vi "OdomLaserSubscriber.vi"() -> (0 "Odom Error Out":errorcluster)   [LabVIEW 2014]
doc: "Reads in the odometry from the Turtlebot"
uses:
  <vilib>/Tufts CEEO ROS for LabVIEW Software/ROS/Code/Console/Servers/ServerSubs/TopicDef.ctl
  <vilib>/Tufts CEEO ROS for LabVIEW Software/ROS/Code/SubVIs/_ROSDirection.ctl
panel:
  out "Scan Details":T1
  in  "?":bool
  in  "Update Time (ms)":u32
  out "Laser Scan Plot (in Husky Frame)":cluster{dbl[], dbl[]}(graph)
  out "Scan Error Out":errorcluster
  out "2D Pose":cluster{"x":dbl, "y":dbl}
  out "Husky Pose Plot":cluster{"X":dbl, "Y":dbl}[](graph)
  out "Husky EKF Odometry":T2
  in  "Stop Subscribing":bool
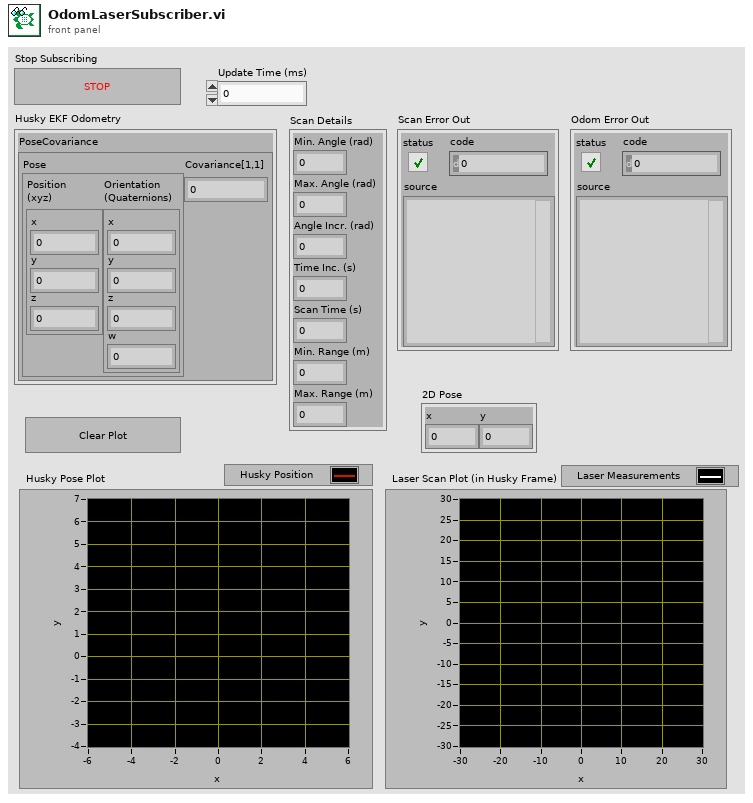
[diagram p1: front panel]
types:
  T1 = cluster{"Min. Angle (rad)":dbl, "Max. Angle (rad)":dbl, "Angle Incr. (rad)":dbl, "Time Inc. (s)":dbl, "Scan Time (s)":dbl, "Min. Range (m)":dbl, "Max. Range (m)":dbl}
  T2 = cluster{"PoseCovariance":cluster{"Pose":cluster{"Position\n(xyz)":cluster{"x":dbl, "y":dbl, "z":dbl}, "Orientation\n(Quaternions)":cluster{"x":dbl, "y":dbl, "z":dbl, "w":dbl}}, "Covariance[1,1]":dbl}}
  T3 = typedef "TopicDef.ctl" = cluster{"Topic":string, "Type":string, "Action":T4, "Update (ms)":u16, "queue size":u16}
  T4 = typedef "_ROSDirection.ctl" = enum16{"Node", "Publisher", "Subscriber", "ServiceClient", "ServiceProvider"}
  T5 = typedef "_ROSControl.ctl" = cluster{"topic port":u16, "Node":string, "topic":string, "type":string, "node port":u16, "error ":errorcluster, "Direction":T4, "Update (ms)":u16, "FIFO size":u16}
  T6 = cluster{"PoseCovariance":cluster{"Pose":cluster{"Point":cluster{"x":dbl, "y":dbl, "z":dbl}, "Quaternion":cluster{"x":dbl, "y":dbl, "z":dbl, "w":dbl}}, "Covariance":dbl}}
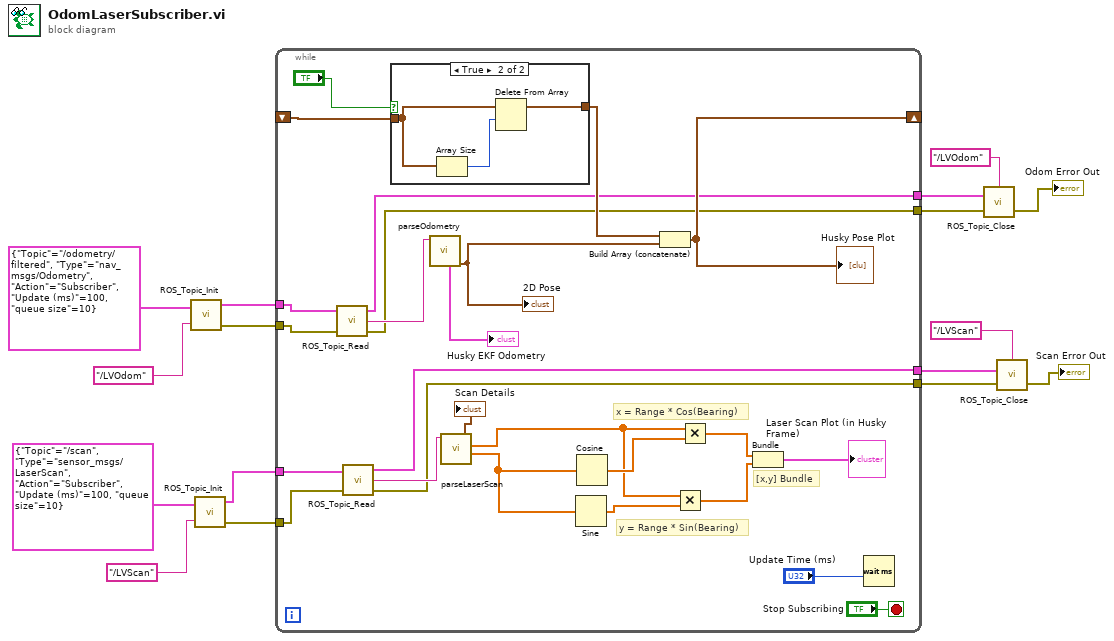
[diagram p0: block diagram]
diagram:
  n1 = call <vilib>:"ROS_Topic_Init.vi"("Definitions"=T3 {"Topic"="/odometry/filtered", "Type"="nav_msgs/Odometry", "Action"=enum."Subscriber", "Update (ms)"=100, "queue size"=10}, "node"="/LVOdom") -> ("ROS out"=w12:T5, "error out"=w11:errorcluster)  [unwired: 1 in]
  n2 = call <vilib>:"ROS_Topic_Init.vi"("Definitions"=T3 {"Topic"="/scan", "Type"="sensor_msgs/LaserScan", "Action"=enum."Subscriber", "Update (ms)"=100, "queue size"=10}, "node"="/LVScan") -> ("ROS out"=w10:T5, "error out"=w9:errorcluster)  [unwired: 1 in]
  n3 = while {
    shift-right: [w41] -> _
    shift-left: _ -> [w24]
    tunnel: w12 -> [w29]
    tunnel: w11 -> [w28]
    tunnel: w10 -> [w27]
    tunnel: w9 -> [w26]
    tunnel: [w20] -> w8
    tunnel: [w19] -> w7
    tunnel: [w18] -> w5
    tunnel: [w17] -> w3
    stop <- "Stop Subscribing" stop-if-true
    # "[x,y] Bundle"
    # "y = Range * Sin(Bearing)"
    # "x = Range * Cos(Bearing)"
    n4 = call <vilib>:"ROS_Topic_Read.vi"("error in (no error)"=w28, "ROS in"=w29) -> ("error out"=w17:errorcluster, "Reply"=w40:string, "ROS out"=w19:T5)  [unwired: 1 in]
    n5 = call <vilib>:"ROS_Topic_Read.vi"("error in (no error)"=w26, "ROS in"=w27) -> ("error out"=w18:errorcluster, "Reply"=w37:string, "ROS out"=w20:T5)  [unwired: 1 in]
    n6 = case shown="True" "?" {
      tunnel: [w43 w45] -> w22
      tunnel: w24 -> [w43 w44]
      frame False {
      }
      frame True {
        n7 = Array Size(array=w44) -> (size(s)=w46:i32)
        n8 = Delete From Array "Delete From Array"(array=w44, length=w46) -> (array with subset deleted=w45:cluster{"x":dbl, "y":dbl}[])  [unwired: 1 in, 1 out]
      }
    }
    n9 = call "parseOdometry.vi"("msg in"=w40) -> ("Odometry"=→"Husky EKF Odometry":T6, "Pose 2D"=w38:cluster{"x":dbl, "y":dbl})  [unwired: 3 in, 3 out]
    "2D Pose" <- w38
    n10 = call "parseLaserScan.vi"("msg in"=w37) -> ("Bearing Array"=w35:dbl[], "Range Array"=w34:sgl[], "Scan Details"=→"Scan Details":T1)  [unwired: 3 in, 1 out]
    n11 = Sine(x=w35) -> (sin(x)=w33:dbl[])
    n12 = Cosine(x=w35) -> (cos(x)=w36:dbl[])
    n13 = Build Array (concatenate)(w22, w38) -> (w41:cluster{"x":dbl, "y":dbl}[])
    "Husky Pose Plot" <- w41
    n14 = Multiply(x=w34, y=w33) -> (x*y=w31:dbl[])
    n15 = Multiply(x=w34, y=w36) -> (x*y=w32:dbl[])
    n16 = Bundle(w32, w31) -> (→"Laser Scan Plot (in Husky Frame)":cluster{dbl[], dbl[]})  [unwired: 1 in]
    n17 = Wait (ms)(milliseconds to wait="Update Time (ms)") -> ()  [unwired: 1 out]
  }
  n18 = call <vilib>:"ROS_Topic_Close.vi"("error in"=w3, "ROS in"=w7, "node"="/LVOdom") -> ("error out"=→"Odom Error Out":errorcluster)  [unwired: 1 in]
  n19 = call <vilib>:"ROS_Topic_Close.vi"("error in"=w5, "ROS in"=w8, "node"="/LVScan") -> ("error out"=→"Scan Error Out":errorcluster)  [unwired: 1 in]
